vi "StripDefectsList.vi"(1 "Defect description list":i32[](array[numeric]), 2 "No of strips":i32, 3 "Bad channel list":i32[](array[numeric])) -> (0 "Defect list":string)   [LabVIEW 2018]
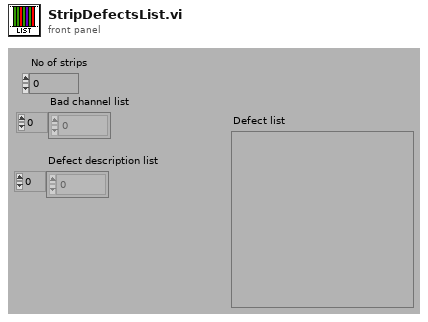
[diagram p1: front panel]
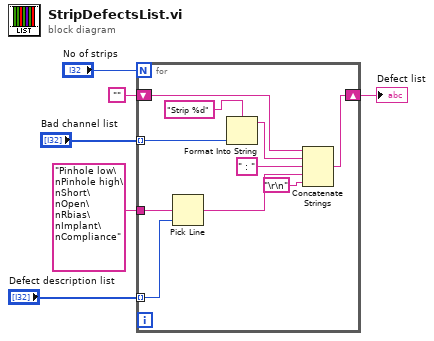
[diagram p0: block diagram]
diagram:
  n1 = for {
    N: "No of strips" -> [_]
    tunnel: "Bad channel list" -> [w7] mode=indexing
    tunnel: "Defect description list" -> [w15] mode=indexing
    tunnel: "Pinhole low\nPinhole high\nShort\nOpen\nRbias\nImplant\nCompliance" -> [w14]
    shift-right: [w12] -> w2
    shift-left: "" -> [w13]
    n2 = Pick Line(multi-line string=w14, line index=w15) -> (output string=w9:string)  [unwired: 1 in]
    n3 = Format Into String(format string="Strip %d", w7) -> (resulting string=w11:string)  [unwired: 2 in, 1 out]
    n4 = Concatenate Strings(w13, w11, " : ", w9, "\r\n") -> (w12:string)
  }
  "Defect list" <- w2
